vi "DOMDefRef.vi"(4 "DOMUserDefRefCommand":T1, 5 "error in (no error)":errorcluster, 6 "Name":string, 8 "Refnum in":refnum<k20>) -> (0 "error out":errorcluster, 2 "Document Session":u64, 3 "Return":i32)   [LabVIEW 2014, in "XML.lvlib"]
uses:
  XML.lvlib
  DOMDefRefCommand.ctl
  DOMUserDefRef.dll
panel:
  out "index of element":i32
  out "Sessions":u64[](array[numeric])
  out "Refs":refnum<k20>[](array[refnum])
  # "Input"
  # "Output"
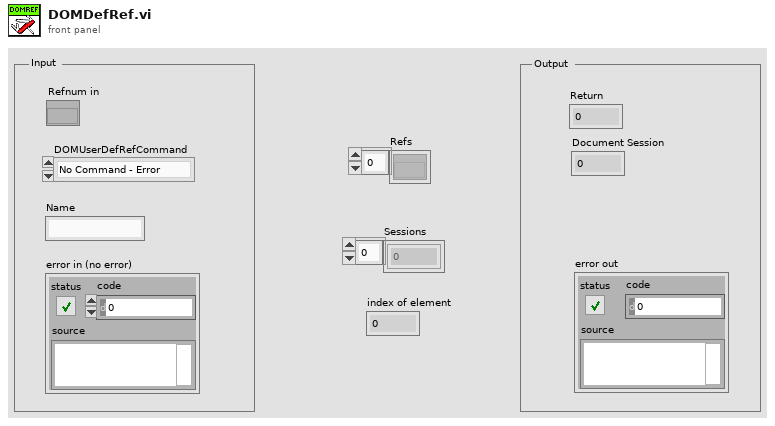
[diagram p1: front panel]
types:
  T1 = typedef "DOMDefRefCommand.ctl" = enum16{"No Command - Error", "Initialise", "Open Document", "Allocate RefNum", "Close Document"}
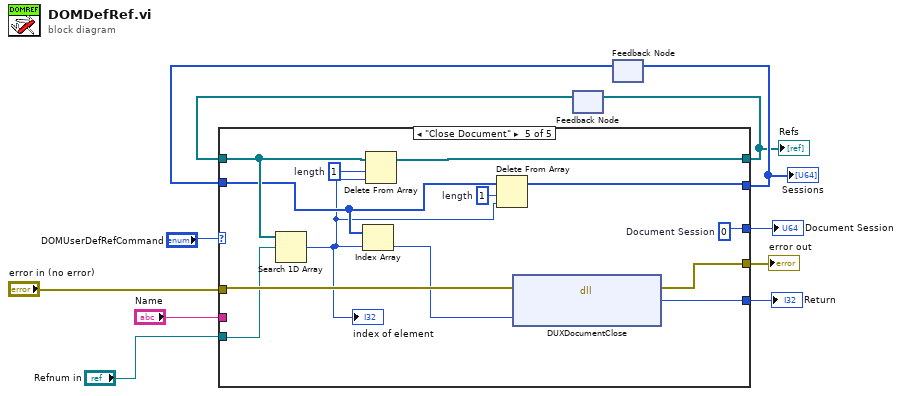
[diagram p0: block diagram]
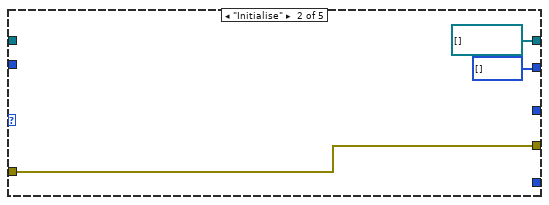
[diagram p3: hidden frame]
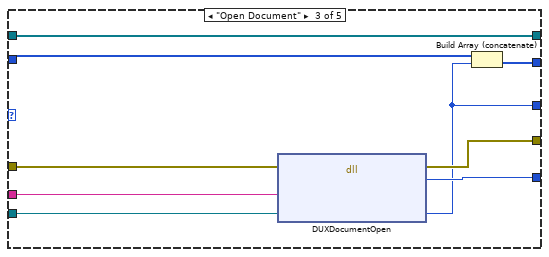
[diagram p4: hidden frame]
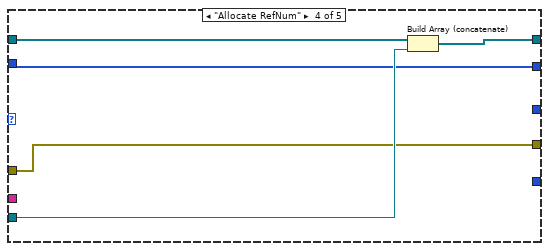
[diagram p5: hidden frame]
diagram:
  n1 = feedback #1() -> (w1:refnum<k20>[])  [unwired: 1 in]
  n2 = feedback #2() -> (w4:u64[])  [unwired: 1 in]
  n3 = case shown="\"Close Document\"" "DOMUserDefRefCommand" {
    tunnel: "Name" -> [_ _ w26 _ _]
    tunnel: [w12 u64[] [] w21 w28 w32] -> w5
    tunnel: [_ _ w25 _ w43] -> w10
    tunnel: [w14 w15 w24 w27 w42] -> w9
    tunnel: "Refnum in" -> [_ _ w23 w31 w40]
    tunnel: "error in (no error)" -> [w14 w15 w22 w27 w44]
    tunnel: w4 -> [w12 _ w20 w28 w35]
    tunnel: [_ _ w19 _ w41] -> w3
    tunnel: [w13 refnum<k20>[] [] w18 w30 w37] -> w2
    tunnel: w1 -> [w13 _ w18 w29 w38]
    frame "No Command - Error", Default {
    }
    frame "Initialise" {
    }
    frame "Open Document" {
      n4 = dll-call lib="DOMUserDefRef.*" fn="DUXDocumentOpen"(error in=w22, "Name"=w26, "Document Session"=w23) -> (error out=w24:errorcluster, "Return"=w25:i32, "Document Session"=w19:u64)  [unwired: 2 in, 2 out]
      n5 = Build Array (concatenate)(w20, w19) -> (w21:u64[])
    }
    frame "Allocate RefNum" {
      n6 = Build Array (concatenate)(w29, w31) -> (w30:refnum<k20>[])
    }
    frame "Close Document" {
      w34 = 1  # length
      w39 = 1  # length
      w41 = u64 0  # Document Session
      n7 = Search 1D Array(1D array=w38, element=w40) -> (index of element=w33:i32)  [unwired: 1 in]
      "index of element" <- w33
      n8 = Index Array(array=w35, index=w33) -> (element=w36:u64)
      n9 = Delete From Array(array=w38, length=w39, index=w33) -> (array with subset deleted=w37:refnum<k20>[])  [unwired: 1 out]
      n10 = Delete From Array(array=w35, length=w34, index=w33) -> (array with subset deleted=w32:u64[])  [unwired: 1 out]
      n11 = dll-call lib="DOMUserDefRef.*" fn="DUXDocumentClose"(error in=w44, "Document Session"=w36) -> (error out=w42:errorcluster, "Return"=w43:i32)  [unwired: 2 in, 2 out]
    }
  }
  "Document Session" <- w3
  "Return" <- w10
  "error out" <- w9
  "Refs" <- w2
  "Sessions" <- w5
  n12 = feedback-in #1(w2) -> ()
  n13 = feedback-in #2(w5) -> ()
